vi "serial_burst_write.vi"(8 "error in (no error)":errorcluster, 10 "Byte array":u16[](array[numeric]) format="%x", 11 "VISA resource name":refnum<visa-resource-name>) -> (0 "error out":errorcluster, 3 "VISA resource name out":refnum<visa-resource-name>)   [LabVIEW 2012]
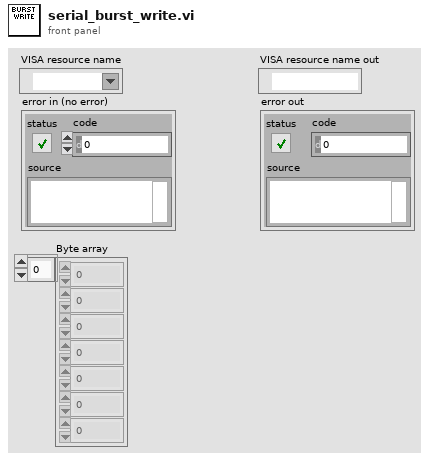
[diagram p1: front panel]
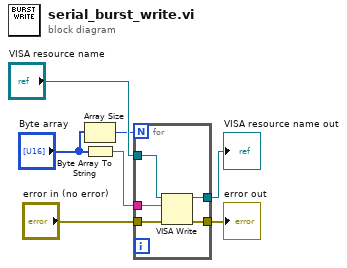
[diagram p0: block diagram]
diagram:
  n1 = Array Size(array="Byte array") -> (size(s)=w3:i32)
  n2 = Byte Array To String(unsigned byte array="Byte array") -> (string=w1:string)
  n3 = for {
    N: w3 -> [_]
    tunnel: "VISA resource name" -> [w12]
    tunnel: "error in (no error)" -> [w11]
    tunnel: [w10] -> w5
    tunnel: [w9] -> w4
    tunnel: w1 -> [w8]
    n4 = VISA Write(VISA resource name=w12, write buffer=w8, error in (no error)=w11) -> (VISA resource name out=w10:refnum<visa-resource-name>, error out=w9:errorcluster)  [unwired: 1 out]
  }
  "VISA resource name out" <- w5
  "error out" <- w4
